vi "Connect To Path.vi"(0 "Power Detector in":refnum<class "Power Detector.lvclass">, 5 "DUT Pin":string, 7 "DUT Site":i32, 11 "error in":errorcluster) -> (4 "Power Detector out":refnum<class "Power Detector.lvclass">, 15 "error out":errorcluster)   [LabVIEW 2023, in "NI Cal-5501 Power Detector.lvlib" / "Power Detector.lvclass"]
uses:
  Power Detector.lvclass
  Common/RFCalAndFixtureCharact.Common.lvlib
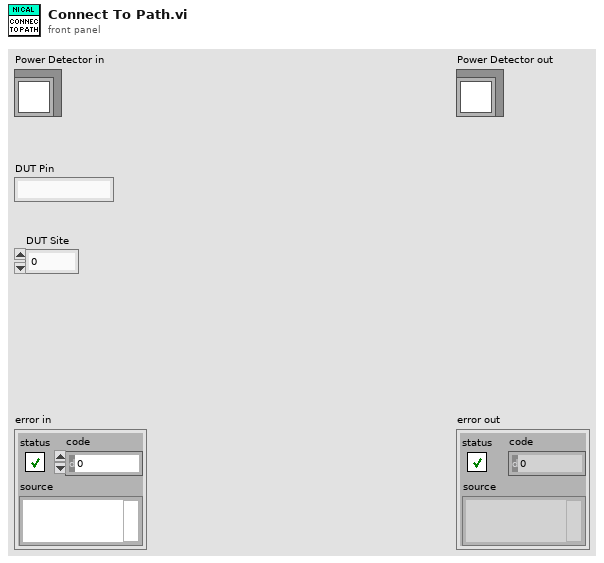
[diagram p1: front panel]
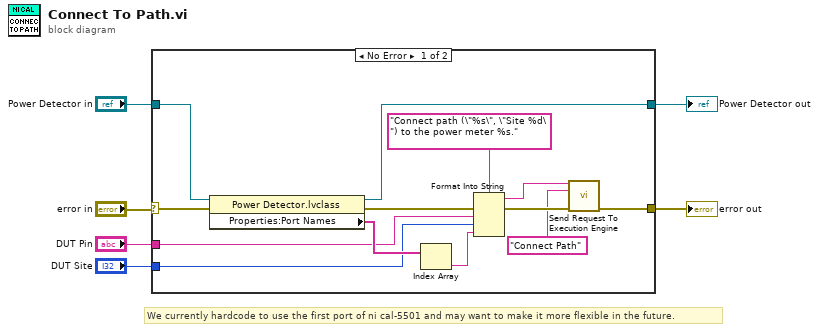
[diagram p0: block diagram]
diagram:
  # "We currently hardcode to use the first port of ni cal-5501 and may want to make it more flexible in the future."
  n1 = case shown="No Error" "error in" {
    selector: "error in" -> [w16 w21]
    tunnel: [w15 w21] -> w3
    tunnel: "Power Detector in" -> [w10 w20]
    tunnel: [w9 w20] -> w4
    tunnel: "DUT Pin" -> [w8 _]
    tunnel: "DUT Site" -> [w7 _]
    frame No Error {
      n2 = property class="Power Detector.lvclass"(reference=w10, error in=w16) -> (reference out=w9:refnum<class "Power Detector.lvclass">, error out=w13:errorcluster, "Properties:Port Names"=w12:string[])
      n3 = Index Array(array=w12) -> (element=w11:string)  [unwired: 1 in]
      n4 = Format Into String(format string="Connect path (\"%s\", \"Site %d\") to the power meter %s." ("message"), error in=w13, w8, w7, w11) -> (resulting string=w18:string, error out=w19:errorcluster)  [unwired: 1 in]
      n5 = call "Send Request To Execution Engine.vi"("Request Message"=w18, "Request Header"="Connect Path", "error in (no error)"=w19) -> ("error out"=w15:errorcluster)  [unwired: 11 in, 1 out]
    }
    frame Error {
    }
  }
  "error out" <- w3
  "Power Detector out" <- w4
